vi "刚度.vi"(6 "关键点2":dbl, 7 "关键点1":dbl, 8 "数组T":dbl[](array[numeric]), 9 "数组D":dbl[](array[numeric])) -> (3 "斜率1":dbl)   [LabVIEW 2013]
uses:
  <vilib>/Analysis/NI_AALPro.lvlib
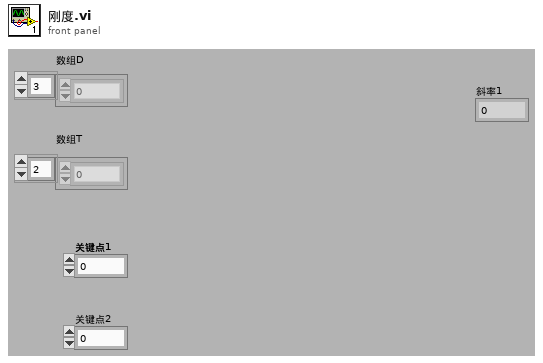
[diagram p1: front panel]
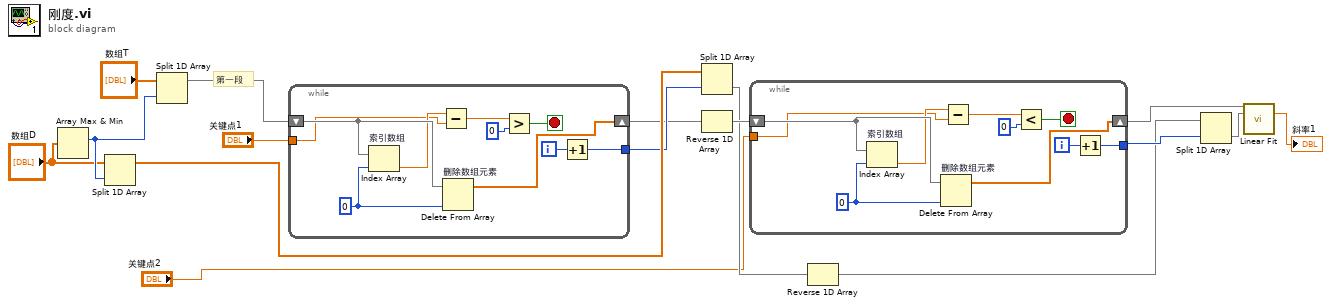
[diagram p0: block diagram]
diagram:
  # "第一段"
  n1 = Array Max & Min(array="数组D") -> (max index (indices)=w16:i32)  [unwired: 3 out]
  n2 = Split 1D Array(array="数组D", index=w16) -> (first subarray=w14:dbl[])  [unwired: 1 out]
  n3 = Split 1D Array(array="数组T", index=w16) -> (first subarray=w15:dbl[])  [unwired: 1 out]
  n4 = while {
    shift-right: [w23] -> w12
    shift-left: w15 -> [w25]
    tunnel: "关键点1" -> [w20]
    tunnel: [w17] -> w13
    i -> [w18]
    stop <- w22 stop-if-true
    w24 = 0
    n5 = Index Array "索引数组"(array=w25, index=w24) -> (element=w21:dbl)
    n6 = Subtract(x=w21, y=w20) -> (x-y=w26:dbl)
    n7 = Delete From Array "删除数组元素"(array=w25, index=w24) -> (array with subset deleted=w23:dbl[])  [unwired: 1 in, 1 out]
    n8 = Greater?(x=w26, y=0) -> (0:w22:bool)
    n9 = Increment(x=w18) -> (x+1=w17:i32)
  }
  n10 = Split 1D Array(array=w14, index=w13) -> (second subarray=w10:dbl[])  [unwired: 1 out]
  n11 = Reverse 1D Array(array=w12) -> (reversed array=w11:dbl[])
  n12 = while {
    shift-right: [w29] -> w4
    shift-left: w11 -> [w35]
    tunnel: "关键点2" -> [w31]
    tunnel: [w27] -> w9
    i -> [w28]
    stop <- w33 stop-if-true
    w34 = 0
    n13 = Index Array "索引数组"(array=w35, index=w34) -> (element=w32:dbl)
    n14 = Delete From Array "删除数组元素"(array=w35, index=w34) -> (array with subset deleted=w29:dbl[])  [unwired: 1 in, 1 out]
    n15 = Subtract(x=w32, y=w31) -> (x-y=w36:dbl)
    n16 = Less?(x=w36, y=0) -> (x < y?=w33:bool)
    n17 = Increment(x=w28) -> (x+1=w27:i32)
  }
  n18 = Reverse 1D Array(array=w10) -> (reversed array=w8:dbl[])
  n19 = Split 1D Array(array=w8, index=w9) -> (second subarray=w5:dbl[])  [unwired: 1 out]
  n20 = call <vilib>:"Linear Fit.vi"("Y"=w4, "X"=w5) -> ("slope"=→"斜率1":dbl)  [unwired: 9 in, 4 out]
